vi "SRV_Sensors - Parse Formula String.vi"(8 "error in (no error)":errorcluster, 11 "Sensor Config":T1 {"Register" format="%.0x"; "I2C Address" format="%.0x"; "Sample Period (ms)" min=10 max=60000 step=1; "Digital Mask" format="%.0x"; "Channel" format="%.0x"}) -> (0 "error out":errorcluster, 1 "Parsed Formula":cluster{"Table":i32[][], "Y Values":dbl[]}, 3 "Sensor Config out":T1 {"Register" format="%.0x"; "I2C Address" format="%.0x"; "Sample Period (ms)" min=10 max=60000 step=1; "Digital Mask" format="%.0x"; "Channel" format="%.0x"})   [LabVIEW 2014]
doc: "Parse formula if not a Digital sensor.\n\n\nAuthor: Mike Schultz (mschultz11711@gmail.com)"
uses:
  SRV_Sensor Config Cluster.ctl
  SRV_Sensor Analog-Digital.ctl
  SRV_Sensor Sampling Mode.ctl
  SRV_Sensor View Config Cluster.ctl
  SRV_Sensors Names.ctl
  SRV_Sensor PicoC Shared Var Type.ctl
  SRV_Sensor Number of Bytes.ctl
  SRV_Sensor Integer Word Type.ctl
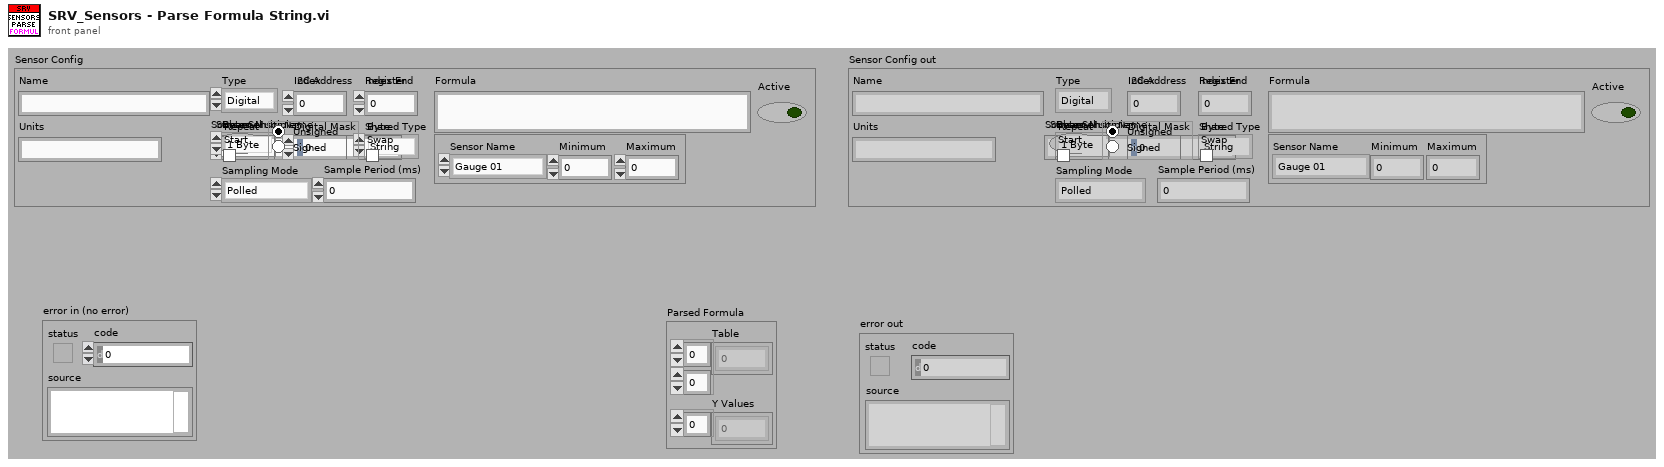
[diagram p1: front panel]
types:
  T1 = typedef "SRV_Sensor Config Cluster.ctl" = cluster{"Name":string, "A/D":T2, "I2C Address":u8, "Register":u8, "Channel":u8, "Digital Mask":u16, "Units":string, "Sampling Mode":T3, "Sample Period (ms)":u32, "Formula":string, "Sensor View Config":T4, "Active":bool, "PicoC Shared Var Type":T6, "Index":u8, "Stream Multiple?":bool, "Index End":u8, "Bytes":T7, "Source Sensor Name":string, "Repeat Start":bool, "Integer Word Type":T8, "Byte Swap":bool}
  T2 = typedef "SRV_Sensor Analog-Digital.ctl" = enum16{"Digital", "Analog", "PicoC Shared", "Calculated"}
  T3 = typedef "SRV_Sensor Sampling Mode.ctl" = enum16{"Polled", "Streaming"}
  T4 = typedef "SRV_Sensor View Config Cluster.ctl" = cluster{"Sensor Name":T5, "Minimum":dbl, "Maximum":dbl}
  T5 = typedef "SRV_Sensors Names.ctl" = enum16{"Gauge 01", "Gauge 02", "Gauge 03", "Gauge 04", "Meter 01", "Meter 02", "Meter 03", "Meter 04", "Numeric 01", "Numeric 02", "Numeric 03", "Numeric 04", "Numeric 05", "Numeric 06", "Numeric 07", "Numeric 08", "Boolean 01", "Boolean 02", "Boolean 03", "Boolean 04", "Boolean 05", "Boolean 06", "Boolean 07", "Boolean 08", "Boolean 09", "Boolean 10", "Boolean 11", "Boolean 12", "Boolean 13", "Boolean 14", "Boolean 15", "Boolean 16", "Boolean 17", "Boolean 18", "Boolean 19", "Boolean 20", "Boolean 21", "Boolean 22", "Boolean 23", "Boolean 24", "Boolean 25", "Boolean 26", "Boolean 27", "Boolean 28", "Boolean 29", "Boolean 30", "Boolean 31", "Boolean 32"}
  T6 = typedef "SRV_Sensor PicoC Shared Var Type.ctl" = enum16{"String", "Integer", "Float"}
  T7 = typedef "SRV_Sensor Number of Bytes.ctl" = enum16{"1 Byte", "2 Bytes"}
  T8 = typedef "SRV_Sensor Integer Word Type.ctl" = enum32{"Unsigned", "Signed"}
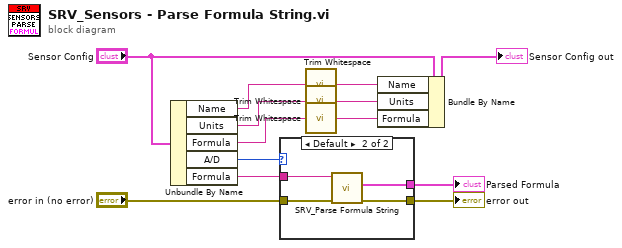
[diagram p0: block diagram]
diagram:
  n1 = Unbundle By Name("Sensor Config") -> ("Name"=w2:string, "Units"=w4:string, "Formula"=w5:string, "A/D"=w9:T2, "Formula"=w12:string)
  n2 = case shown="Default" w9 {
    tunnel: [_ w18] -> w13
    tunnel: w12 -> [_ w17]
    tunnel: [w14 w16] -> w11
    tunnel: "error in (no error)" -> [w14 w15]
    frame "Digital" {
    }
    frame Default {
      n3 = call "SRV_Parse Formula String.vi"("error in (no error)"=w15, "Formula"=w17) -> ("error out"=w16:errorcluster, "Parsed Formula"=w18:cluster{"Table":i32[][], "Y Values":dbl[]})  [unwired: 8 in]
    }
  }
  "Parsed Formula" <- w13
  "error out" <- w11
  n4 = call <vilib>:"Trim Whitespace.vi"("string"=w2) -> ("trimmed string"=w1:string)  [unwired: 1 in]
  n5 = call <vilib>:"Trim Whitespace.vi"("string"=w4) -> ("trimmed string"=w3:string)  [unwired: 1 in]
  n6 = call <vilib>:"Trim Whitespace.vi"("string"=w5) -> ("trimmed string"=w6:string)  [unwired: 1 in]
  n7 = Bundle By Name(cluster="Sensor Config", "Name"=w1, "Units"=w3, "Formula"=w6) -> (→"Sensor Config out":T1)
